vi "startDio64.vi"(8 "error in (no error)":errorcluster, 11 "BECHWCBasic in":refnum<class "BECHWCBasic.lvclass">) -> (0 "error out":errorcluster, 3 "BECHWCBasic out":refnum<class "BECHWCBasic.lvclass">)   [LabVIEW 2009, in "Hardware.lvlib" / "HWControllers.lvlib" / "BECHWCBasic.lvclass"]
doc: "Start the DIO64 timing card"
uses:
  BECHWCBasic.lvclass
  BECHWCBasic.lvclass/BECHWCBasic.ctl
  Channels/Digital/DigitalOutput.lvclass
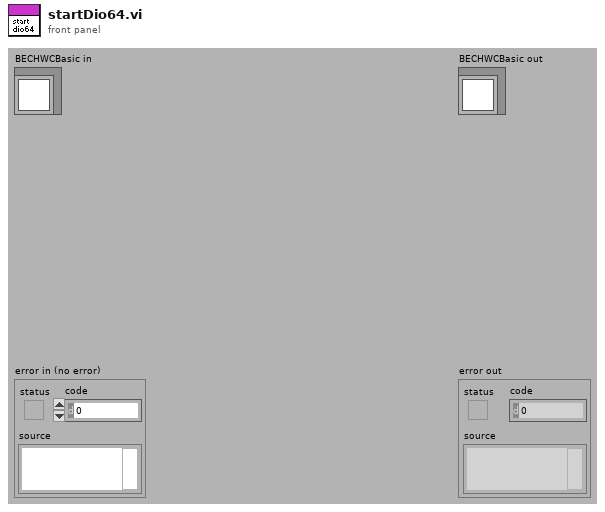
[diagram p1: front panel]
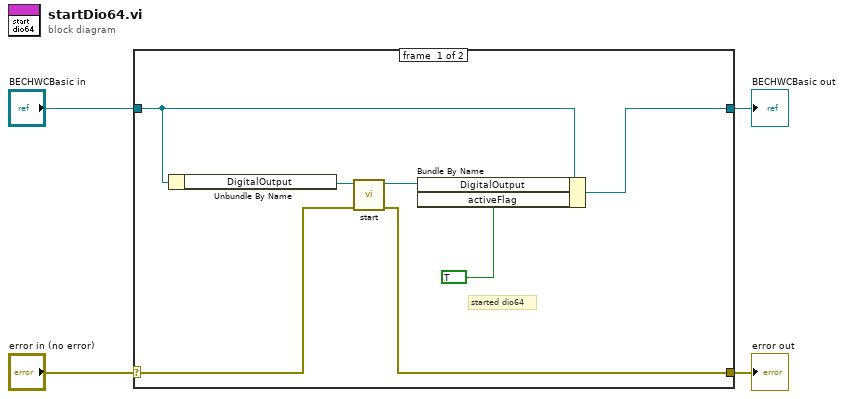
[diagram p0: block diagram]
diagram:
  n1 = case shown="No Error" "error in (no error)" {
    selector: "error in (no error)" -> [w7 w13]
    tunnel: [w6 w13] -> w3
    tunnel: [w8 w12] -> w1
    tunnel: "BECHWCBasic in" -> [w9 w12]
    frame #0 {
      # "started dio64"
      n2 = Unbundle By Name(w9) -> ("DigitalOutput"=w11:refnum<class "DigitalOutput.lvclass">)
      n3 = call-dynamic "start.vi"("error in (no error)"=w7, "DigitalOutput in"=w11) -> ("error out"=w6:errorcluster, "DigitalOutput out"=w10:refnum<class "DigitalOutput.lvclass">)  [unwired: 8 in]
      n4 = Bundle By Name(cluster=w9, "DigitalOutput"=w10, "activeFlag"=TRUE) -> (w8:refnum<class "BECHWCBasic.lvclass">)
    }
    frame #1 {
    }
  }
  "error out" <- w3
  "BECHWCBasic out" <- w1
